vi "PBar-Start Indeterminate.vi"(0 "Slide":refnum<vi>, 7 "Caption.Text":string="Running script", 11 "error in (no error)":errorcluster) -> (4 "reference out":refnum<vi>, 15 "error out":errorcluster)   [LabVIEW 2020]
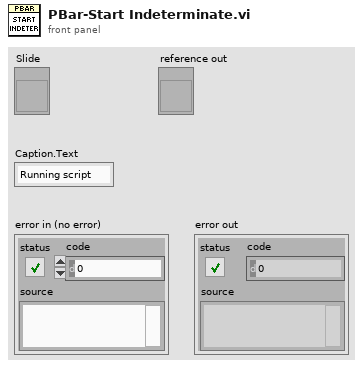
[diagram p1: front panel]
types:
  T1 = enum32{"Invalid", "Standard", "Closed", "Hidden", "Minimized", "Maximized"}
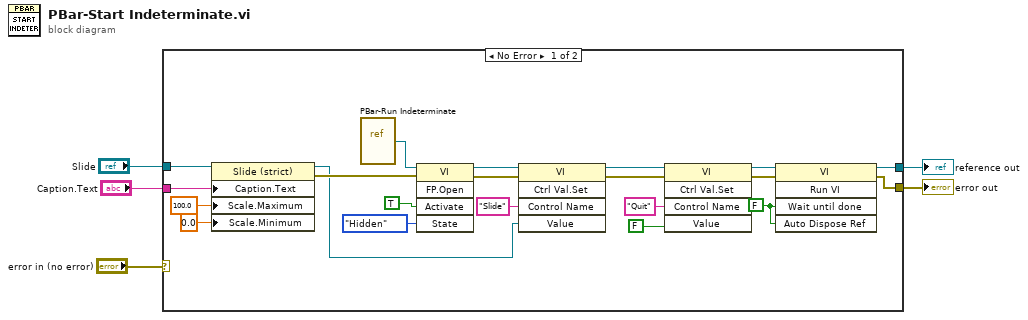
[diagram p0: block diagram]
diagram:
  n1 = case shown="No Error" "error in (no error)" {
    selector: "error in (no error)" -> [_ w27]
    tunnel: "Caption.Text" -> [w26 _]
    tunnel: "Slide" -> [w25 _]
    tunnel: [w14 _] -> w3
    tunnel: [w7 w27] -> w1
    frame No Error {
      w23 = FALSE ("Wait Until Done")
      n2 = property class="Slide (strict)"(reference=w25, "Caption.Text"=w26, "Scale.Maximum"=100.0 ("y"), "Scale.Minimum"=0.0 ("Scale.Range:Minimum")) -> (reference out=w15:refnum<vi>, error out=w19:errorcluster)  [unwired: 1 in]
      n3 = vi-ref "PBar-Run Indeterminate.vi"() -> (w21:refnum<vi>)
      n4 = invoke class="VI" method="FP.Open"(reference=w21, error in=w19, "Activate"=TRUE ("Activate?"), "State"=T1."Hidden") -> (reference out=w18:refnum<vi>, error out=w17:errorcluster)  [unwired: 1 in, 3 out]
      n5 = invoke class="VI" method="Ctrl Val.Set"(reference=w18, error in=w17, "Control Name"="Slide", "Value"=w15) -> (reference out=w12:refnum<vi>, error out=w11:errorcluster)  [unwired: 1 in, 3 out]
      n6 = invoke class="VI" method="Ctrl Val.Set"(reference=w12, error in=w11, "Control Name"="Quit", "Value"=FALSE) -> (reference out=w10:refnum<vi>, error out=w9:errorcluster)  [unwired: 1 in, 3 out]
      n7 = invoke class="VI" method="Run VI"(reference=w10, error in=w9, "Wait until done"=w23, "Auto Dispose Ref"=w23) -> (reference out=w14:refnum<vi>, error out=w7:errorcluster)  [unwired: 1 in, 3 out]
    }
    frame Error {
    }
  }
  "reference out" <- w3
  "error out" <- w1
